vi "multiple_counters.vi"() -> ()   [LabVIEW 2010]
doc: "This example demonstrates how to generate a finite number of digital pulses using a counter output.\n\nOn some hardware, this requires the use of a second counter to generate a gate signal. If necessary, DAQmx configures this second counter for you."
uses:
  <libdir>/resource/objmgr/daqmx.rc
  <vilib>/DAQmx/configure/timing.llb/DAQmx Timing (Implicit).vi
  <vilib>/DAQmx/configure/trigger.llb/DAQmx Start Trigger (Digital Edge).vi
  <vilib>/Utility/error.llb/DialogType.ctl
  <vilib>/DAQmx/create/channels.llb/DAQmx Create Channel (CO-Pulse Generation-Time).vi
  <vilib>/DAQmx/create/channels.llb/DAQmx Create Channel (CO-Pulse Generation-Frequency).vi
panel:
  in  "Stop 4":bool
  in  "high time 4":dbl=0.01 format="%.6f"
  in  "low time 4":dbl=0.01 format="%.6f"
  in  "initial delay 4":dbl format="%.6f"
  in  "Number of Pulses 4":i32=1000
  in  "Output Terminal 4":tag="/Dev1/PFI12"
  in  "Counter 4":tag="Dev1/ctr0"
  in  "Stop 3":bool
  in  "Stop 2":bool
  in  "high time 2":dbl=0.01 format="%.6f"
  in  "low time 2":dbl=0.01 format="%.6f"
  in  "high time 3":dbl=0.01 format="%.6f"
  in  "low time 3":dbl=0.01 format="%.6f"
  in  "initial delay 3":dbl format="%.6f"
  in  "initial delay 2":dbl format="%.6f"
  in  "Number of Pulses 3":i32=1000
  in  "Output Terminal 3":tag="/Dev1/PFI12"
  in  "Counter 3":tag="Dev1/ctr0"
  in  "Number of Pulses 2":i32=1000
  in  "Output Termina 2":tag="/Dev1/PFI12"
  in  "Counter 2":tag="Dev1/ctr0"
  # "Trigger Control Panel"
  # "HV Trigger"
  # "Amp Trigger"
  # "Laser Trigger"
  # "Channel 2 Settings"
  # "Channel 3 Settings"
  # "Channel 4 Settings"
  # "Timing Settings"
  # "Timing Settings"
  # "Timing Settings"
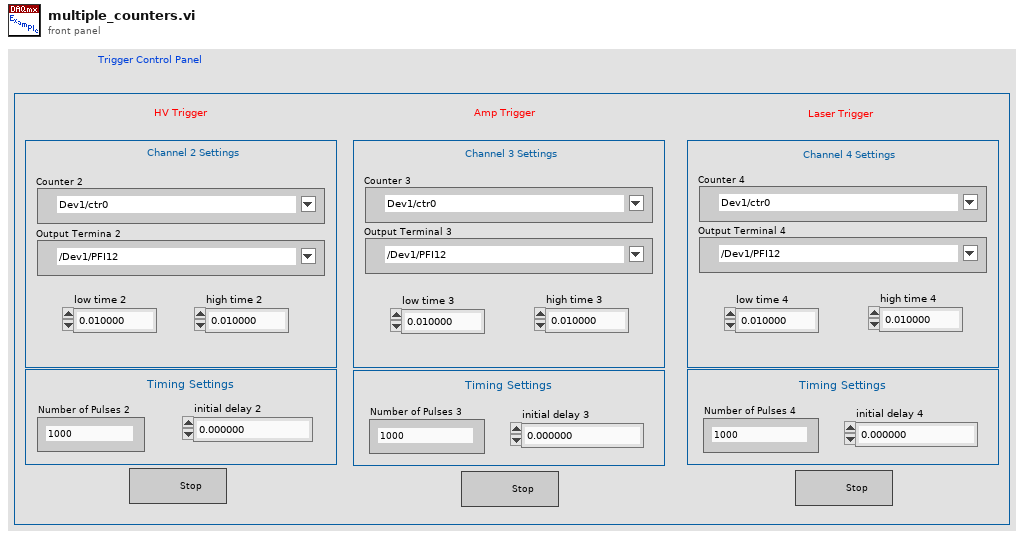
[diagram p1: front panel]
types:
  T1 = typedef "DialogType.ctl" = u16
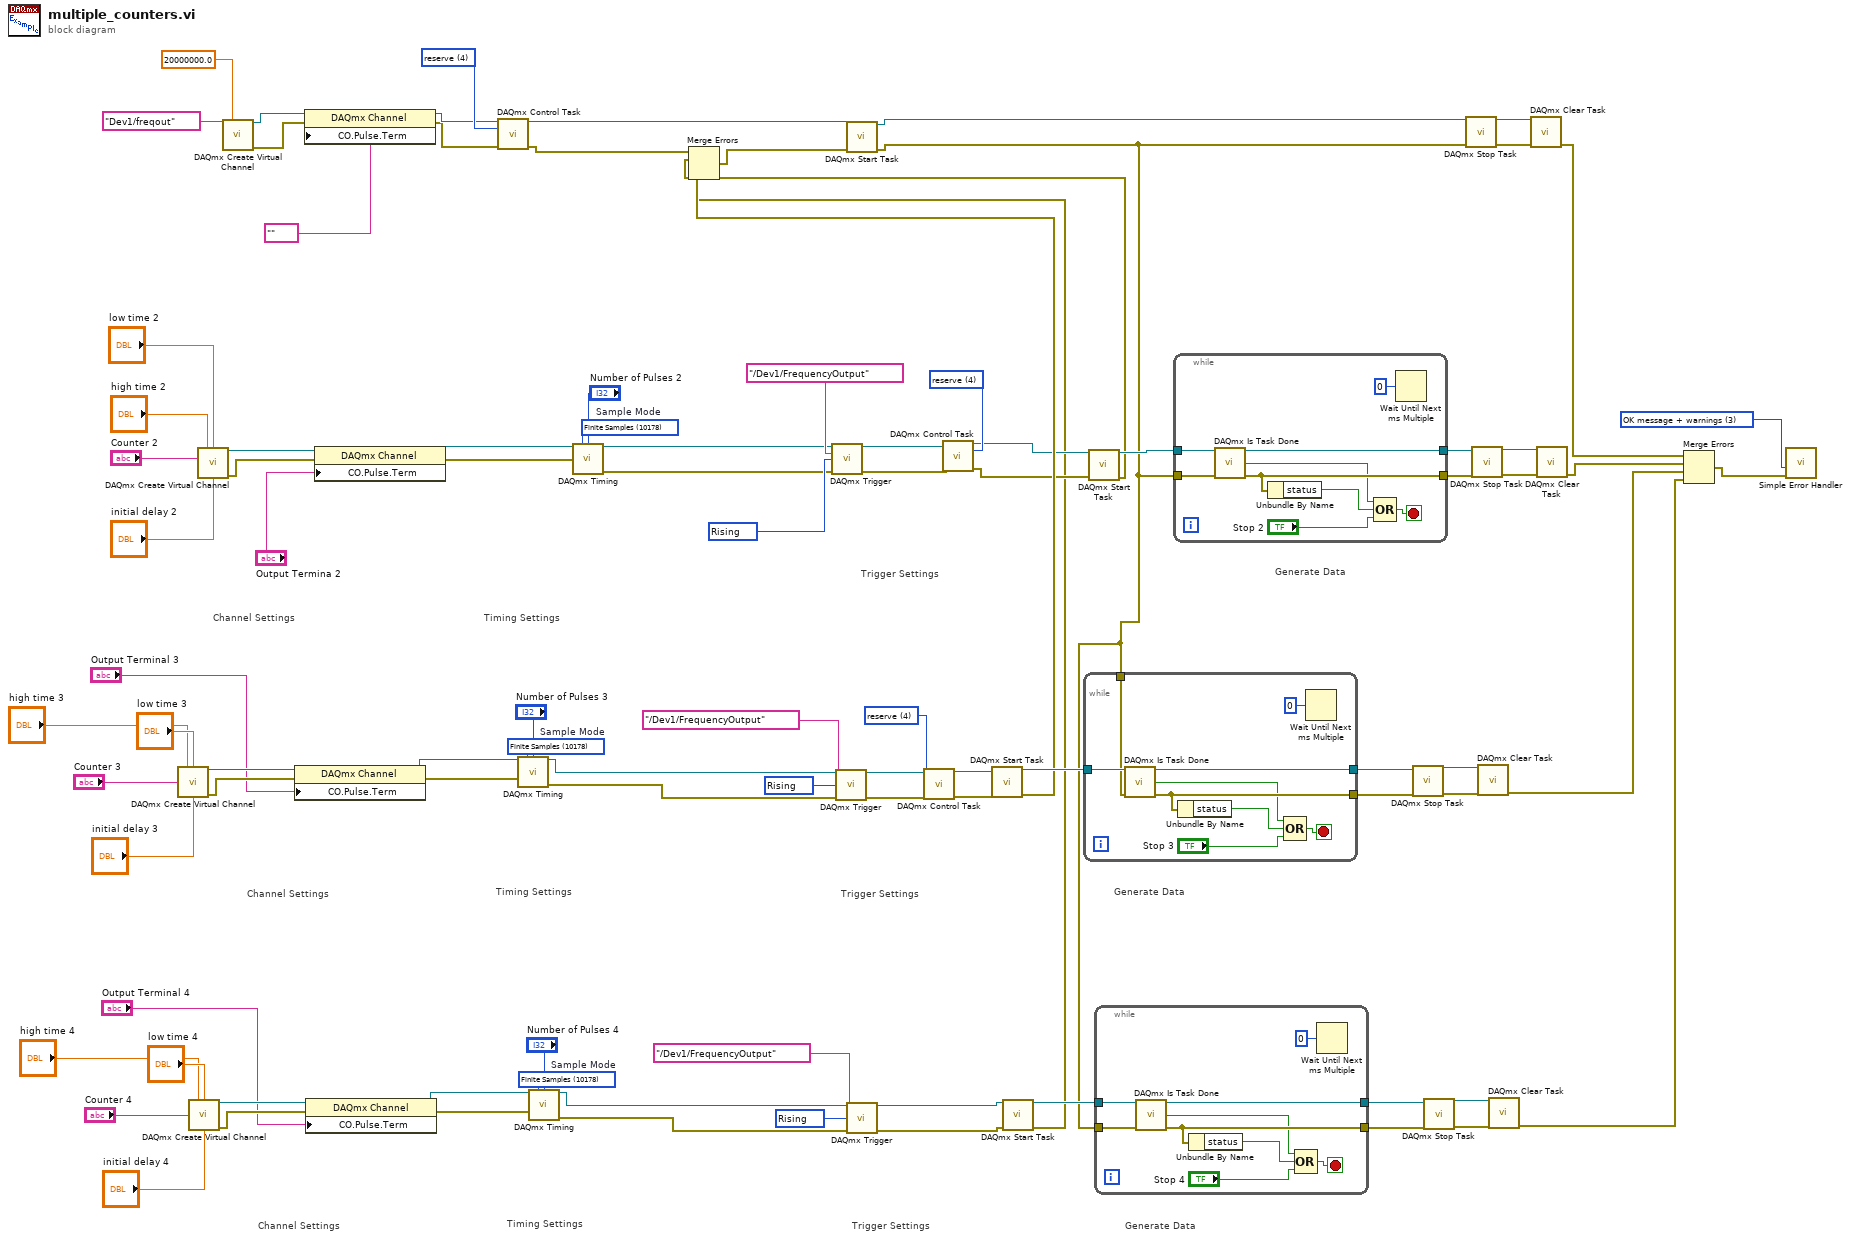
[diagram p0: block diagram]
diagram:
  w4 = 4 items=["verify"=2, "reserve"=4, "commit"=3, "unreserve"=5, "abort"=6] ("action")
  w13 = 10280 items=["Rising"=10280, "Falling"=10171] ("edge")
  w30 = 10178 items=["Finite Samples"=10178, "Continuous Samples"=10123, "Hardware Timed Single Point"=12522]  # Sample Mode
  w39 = 10280 items=["Rising"=10280, "Falling"=10171] ("edge")
  w41 = 4 items=["verify"=2, "reserve"=4, "commit"=3, "unreserve"=5, "abort"=6] ("action")
  w44 = 10280 items=["Rising"=10280, "Falling"=10171] ("edge")
  w67 = 4 items=["verify"=2, "reserve"=4, "commit"=3, "unreserve"=5, "abort"=6] ("action")
  w85 = 10178 items=["Finite Samples"=10178, "Continuous Samples"=10123, "Hardware Timed Single Point"=12522]  # Sample Mode
  w86 = T1 3 items=["no dialog", "OK message", "continue or stop message", "OK message + warnings", "continue/stop + warnings"] ("type of dialog (OK msg:1)")
  w96 = 10178 items=["Finite Samples"=10178, "Continuous Samples"=10123, "Hardware Timed Single Point"=12522]  # Sample Mode
  # "Generate Data"
  # "Trigger Settings"
  # "Timing Settings"
  # "Channel Settings"
  # "Generate Data"
  # "Generate Data"
  # "Trigger Settings"
  # "Timing Settings"
  # "Channel Settings"
  # "Trigger Settings"
  # "Timing Settings"
  # "Channel Settings"
  n1 = call-poly <vilib>:"DAQmx Create Virtual Channel.vi"("high time"="high time 3", "low time"="low time 3", "counter"="Counter 3", "initial delay"="initial delay 3") -> ("task out"=w83:refnum<k21>, "error out"=w82:errorcluster)  [unwired: 10 in]
  n2 = call-poly <vilib>:"DAQmx Create Virtual Channel.vi"("high time"="high time 4", "low time"="low time 4", "counter"="Counter 4", "initial delay"="initial delay 4") -> ("task out"=w28:refnum<k21>, "error out"=w27:errorcluster)  [unwired: 10 in]
  n3 = call-poly <vilib>:"DAQmx Create Virtual Channel.vi"("high time"="high time 2", "low time"="low time 2", "counter"="Counter 2", "initial delay"="initial delay 2") -> ("task out"=w94:refnum<k21>, "error out"=w93:errorcluster)  [unwired: 10 in]
  n4 = call-poly <vilib>:"DAQmx Create Virtual Channel.vi"("frequency"=20000000.0, "counter"=tag "Dev1/freqout") -> ("task out"=w48:refnum<k21>, "error out"=w47:errorcluster)  [unwired: 12 in]
  n5 = property class="DAQmx Channel"(reference=w83, error in=w82, "CO.Pulse.Term"="Output Terminal 3") -> (reference out=w79:refnum<k21>, error out=w80:errorcluster)
  n6 = property class="DAQmx Channel"(reference=w48, error in=w47, "CO.Pulse.Term"=tag "") -> (reference out=w50:refnum<k21>, error out=w49:errorcluster)
  n7 = property class="DAQmx Channel"(reference=w28, error in=w27, "CO.Pulse.Term"="Output Terminal 4") -> (reference out=w24:refnum<k21>, error out=w25:errorcluster)
  n8 = property class="DAQmx Channel"(reference=w94, error in=w93, "CO.Pulse.Term"="Output Termina 2") -> (reference out=w90:refnum<k21>, error out=w91:errorcluster)
  n9 = call <vilib>:"DAQmx Control Task.vi"("task/channels in"=w50, "action"=w67, "error in"=w49) -> ("task out"=w68:refnum<k21>, "error out"=w66:errorcluster)  [unwired: 11 in]
  n10 = call-poly <vilib>:"DAQmx Timing.vi"("task/channels in"=w79, "sample mode"=w85, "samples per channel"="Number of Pulses 3", "error in"=w80) -> ("task out"=w43:refnum<k21>, "error out"=w42:errorcluster)  [unwired: 10 in]
  n11 = call-poly <vilib>:"DAQmx Timing.vi"("task/channels in"=w24, "sample mode"=w30, "samples per channel"="Number of Pulses 4", "error in"=w25) -> ("task out"=w10:refnum<k21>, "error out"=w9:errorcluster)  [unwired: 10 in]
  n12 = call-poly <vilib>:"DAQmx Timing.vi"("task/channels in"=w90, "sample mode"=w96, "samples per channel"="Number of Pulses 2", "error in"=w91) -> ("task out"=w36:refnum<k21>, "error out"=w35:errorcluster)  [unwired: 10 in]
  n13 = call-poly <vilib>:"DAQmx Trigger.vi"("task/channels in"=w36, "source"=tag "/Dev1/FrequencyOutput", "edge"=w39, "error in"=w35) -> ("task out"=w38:refnum<k21>, "error out"=w40:errorcluster)  [unwired: 10 in]
  n14 = call-poly <vilib>:"DAQmx Trigger.vi"("task/channels in"=w43, "source"=tag "/Dev1/FrequencyOutput", "edge"=w44, "error in"=w42) -> ("task out"=w8:refnum<k21>, "error out"=w7:errorcluster)  [unwired: 10 in]
  n15 = call-poly <vilib>:"DAQmx Trigger.vi"("task/channels in"=w10, "source"=tag "/Dev1/FrequencyOutput", "edge"=w13, "error in"=w9) -> ("task out"=w12:refnum<k21>, "error out"=w11:errorcluster)  [unwired: 10 in]
  n16 = call <vilib>:"DAQmx Control Task.vi"("task/channels in"=w8, "action"=w4, "error in"=w7) -> ("task out"=w6:refnum<k21>, "error out"=w5:errorcluster)  [unwired: 11 in]
  n17 = call <vilib>:"DAQmx Control Task.vi"("task/channels in"=w38, "action"=w41, "error in"=w40) -> ("task out"=w34:refnum<k21>, "error out"=w33:errorcluster)  [unwired: 11 in]
  n18 = call <vilib>:"DAQmx Start Task.vi"("task/channels in"=w6, "error in"=w5) -> ("task out"=w64:refnum<k21>, "error out"=w58:errorcluster)  [unwired: 12 in]
  n19 = call <vilib>:"DAQmx Start Task.vi"("task/channels in"=w12, "error in"=w11) -> ("task out"=w17:refnum<k21>, "error out"=w3:errorcluster)  [unwired: 12 in]
  n20 = call <vilib>:"DAQmx Start Task.vi"("task/channels in"=w34, "error in"=w33) -> ("task out"=w65:refnum<k21>, "error out"=w59:errorcluster)  [unwired: 12 in]
  n21 = Merge Errors(w66, w59, w58, w3) -> (w57:errorcluster)
  n22 = call <vilib>:"DAQmx Start Task.vi"("task/channels in"=w68, "error in"=w57) -> ("task out"=w54:refnum<k21>, "error out"=w2:errorcluster)  [unwired: 12 in]
  n23 = while {
    tunnel: w64 -> [w105]
    tunnel: [w102] -> w60
    tunnel: [w103] -> w61
    tunnel: w2 -> [w97]
    stop <- w104 stop-if-true
    n24 = call <vilib>:"DAQmx Is Task Done.vi"("task/channels in"=w105, "error in"=w97) -> ("task out"=w103:refnum<k21>, "task done?"=w98:bool, "error out"=w102:errorcluster)  [unwired: 11 in]
    n25 = Unbundle By Name(w102) -> ("status"=w101:bool)
    n26 = Compound Arithmetic op=OR(w98, w101, "Stop 3") -> (w104:bool)
    n27 = Wait Until Next ms Multiple(millisecond multiple=u32 0) -> ()  [unwired: 1 out]
  }
  n28 = while {
    tunnel: w17 -> [w114]
    tunnel: [w111] -> w15
    tunnel: [w112] -> w16
    tunnel: w2 -> [w106]
    stop <- w113 stop-if-true
    n29 = call <vilib>:"DAQmx Is Task Done.vi"("task/channels in"=w114, "error in"=w106) -> ("task out"=w112:refnum<k21>, "task done?"=w107:bool, "error out"=w111:errorcluster)  [unwired: 11 in]
    n30 = Unbundle By Name(w111) -> ("status"=w110:bool)
    n31 = Compound Arithmetic op=OR(w107, w110, "Stop 4") -> (w113:bool)
    n32 = Wait Until Next ms Multiple(millisecond multiple=u32 0) -> ()  [unwired: 1 out]
  }
  n33 = while {
    tunnel: w65 -> [w123]
    tunnel: [w120] -> w62
    tunnel: [w121] -> w63
    tunnel: w2 -> [w115]
    stop <- w122 stop-if-true
    n34 = call <vilib>:"DAQmx Is Task Done.vi"("task/channels in"=w123, "error in"=w115) -> ("task out"=w121:refnum<k21>, "task done?"=w116:bool, "error out"=w120:errorcluster)  [unwired: 11 in]
    n35 = Unbundle By Name(w120) -> ("status"=w119:bool)
    n36 = Compound Arithmetic op=OR(w116, w119, "Stop 2") -> (w122:bool)
    n37 = Wait Until Next ms Multiple(millisecond multiple=u32 0) -> ()  [unwired: 1 out]
  }
  n38 = call <vilib>:"DAQmx Stop Task.vi"("task/channels in"=w61, "error in"=w60) -> ("task out"=w77:refnum<k21>, "error out"=w76:errorcluster)  [unwired: 12 in]
  n39 = call <vilib>:"DAQmx Stop Task.vi"("task/channels in"=w16, "error in"=w15) -> ("task out"=w22:refnum<k21>, "error out"=w21:errorcluster)  [unwired: 12 in]
  n40 = call <vilib>:"DAQmx Stop Task.vi"("task/channels in"=w54, "error in"=w2) -> ("task out"=w56:refnum<k21>, "error out"=w55:errorcluster)  [unwired: 12 in]
  n41 = call <vilib>:"DAQmx Stop Task.vi"("task/channels in"=w63, "error in"=w62) -> ("task out"=w88:refnum<k21>, "error out"=w87:errorcluster)  [unwired: 12 in]
  n42 = call <vilib>:"DAQmx Clear Task.vi"("task in"=w77, "error in"=w76) -> ("error out"=w53:errorcluster)  [unwired: 13 in]
  n43 = call <vilib>:"DAQmx Clear Task.vi"("task in"=w22, "error in"=w21) -> ("error out"=w1:errorcluster)  [unwired: 13 in]
  n44 = call <vilib>:"DAQmx Clear Task.vi"("task in"=w56, "error in"=w55) -> ("error out"=w31:errorcluster)  [unwired: 13 in]
  n45 = call <vilib>:"DAQmx Clear Task.vi"("task in"=w88, "error in"=w87) -> ("error out"=w32:errorcluster)  [unwired: 13 in]
  n46 = Merge Errors(w31, w32, w53, w1) -> (w52:errorcluster)
  n47 = call <vilib>:"Simple Error Handler.vi"("type of dialog (OK msg:1)"=w86, "error in (no error)"=w52) -> ()  [unwired: 3 in, 5 out]
